vi "Actor Core.vi"(8 "error in":errorcluster, 11 "Nested in":refnum<class "ViewController.lvclass">) -> (0 "error out":errorcluster, 3 "Actor out":refnum<class "Actor.lvclass">)   [LabVIEW 2015, in "ViewController.lvlib" / "ViewController.lvclass"]
doc: "(<B>Filename</B>: Actor Framework.lvlib:Actor.lvclass:Actor Core.vi)\n\nReceives messages to the actor, reacts to them, and initiates any error handling that may shut the actor down.\n\nDescendant classes may override this VI to append parallel tasks for the actor to complete while it handles messages. Overrides use the Call Parent Method node."
uses:
  ViewController.lvclass
  <vilib>/ActorFramework/Actor/Actor.lvclass
  <vilib>/ActorFramework/Stop Msg/Stop Msg.lvclass
  Interface Messages/VI Infomation RTM Msg/VI Infomation RTM Msg.lvclass
  Interface/Interface.lvclass
  Interface Messages/VI Information Change Msg/VI Information Change Msg.lvclass
  Interface/Controls/VI Infomation.ctl
  Interface/Interface.lvlib
panel:
  in  "VI Information":T1[](array[typedef])
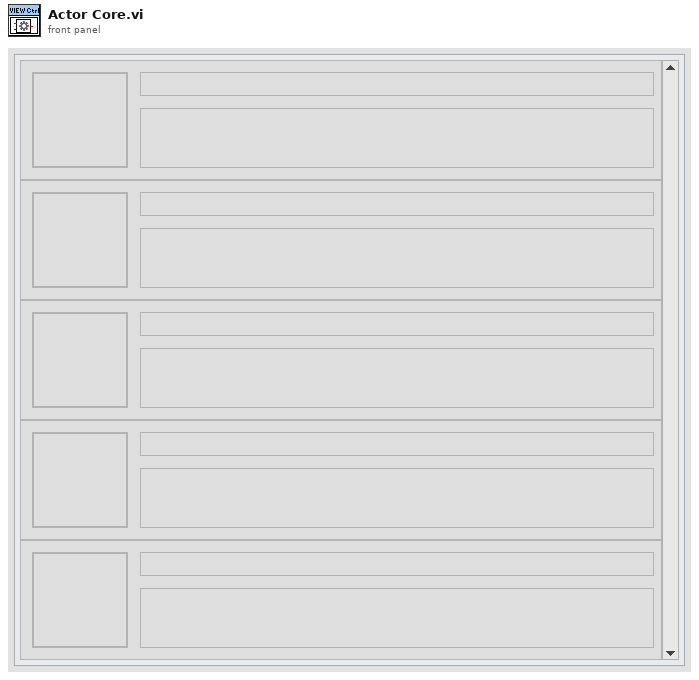
[diagram p1: front panel]
types:
  T1 = typedef "Interface.lvlib/VI Infomation.ctl" = cluster{"VI Name":string, "VI Description":string, "VI Icon":picture}
  T2 = enum8{"Enabled", "Disabled", "Disabled and Grayed Out"}
  T3 = cluster{"Stop":refnum<user-event>, "VI Infomation":refnum<user-event>}
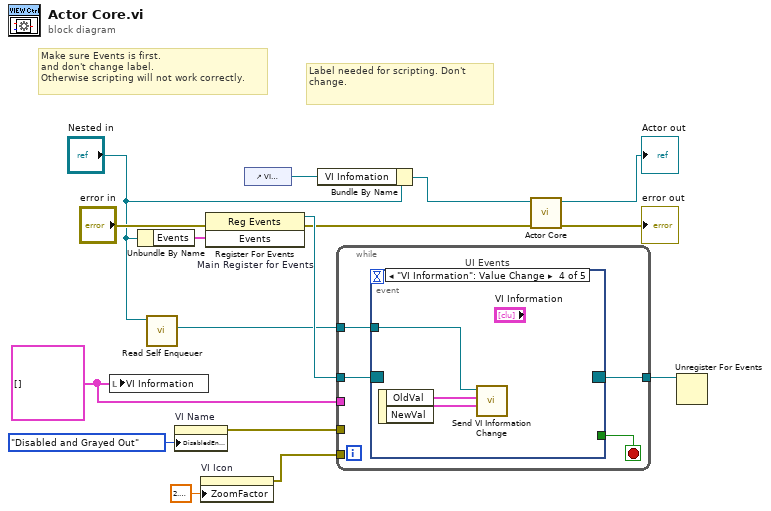
[diagram p0: block diagram]
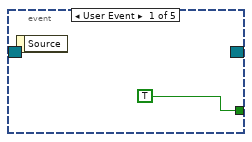
[diagram p2: hidden frame]
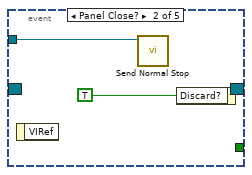
[diagram p3: hidden frame]
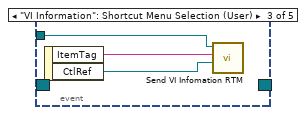
[diagram p4: hidden frame]
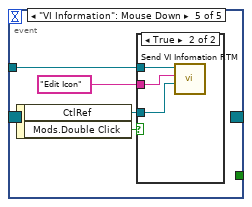
[diagram p5: hidden frame]
diagram:
  w3 = T1[] [] ("VI Information")
  # "Label needed for scripting. Don't change."
  # "Make sure Events is first.\nand don't change label.\nOtherwise scripting will not work correctly."
  n1 = local write "VI Information"(w3) -> ()
  n2 = Unbundle By Name("Nested in") -> ("Events"=w13:T3)
  n3 = call <vilib>:"Read Self Enqueuer.vi"("Actor"="Nested in") -> ("Self Enqueuer"=w11:refnum<class "Message Enqueuer.lvclass">)  [unwired: 10 in]
  n4 = property on="VI Name" class="Str"("DisabledEnum"=T2."Disabled and Grayed Out" ("Disabled")) -> (error out=w7:errorcluster)  [unwired: 2 in, 1 out]
  n5 = property on="VI Icon" class="Pict"("ZoomFactor"=sgl 2.9 ("Zoom Factor")) -> (error out=w1:errorcluster)  [unwired: 2 in, 1 out]
  n6 = register-events "Main Register for Events"(error in="error in", w13) -> (reference out=w14:refnum<event-registration>, error out=w9:errorcluster)  [unwired: 1 in]
  n7 = control-ref of="VI Information"() -> (w6:refnum<vi>)
  n8 = Bundle By Name(cluster="Nested in", "VI Infomation"=w6) -> (w4:refnum<class "ViewController.lvclass">)
  n9 = while {
    tunnel: w14 -> [w20]
    tunnel: [w18] -> w12
    tunnel: w11 -> [w17]
    tunnel: w7 -> [_]
    tunnel: w3 -> [_]
    tunnel: w1 -> [_]
    stop <- w19 stop-if-true
    n10 = event "UI Events" shown="[3] \"VI Information\": Value Change" {
      selector: w20 -> [_ _ _ _ _]
      dyn-events: [_ _ _ _ _] -> w18
      timeout: _ -> [_ _ _ _ _]
      tunnel: [TRUE _ _ _ _] -> w19
      tunnel: w17 -> [_ w22 w24 w29 w32]
      event User Event {
        n11 = event-data() -> ()  [unwired: 1 in, 1 out]
      }
      event Panel Close? {
        n12 = event-data() -> ()  [unwired: 1 in, 1 out]
        n13 = call <vilib>:"Send Normal Stop.vi"("Message Enqueuer"=w22) -> ()  [unwired: 10 in, 1 out]
        n14 = event-data("Discard?"=TRUE) -> ()  [unwired: 1 in, 1 out]
      }
      event "VI Information": Shortcut Menu Selection (User) {
        n15 = event-data() -> ("ItemTag"=w26:string, "CtlRef"=w25:refnum<vi>)  [unwired: 1 in]
        n16 = call "Send VI Infomation RTM.vi"("Ctl Refnum"=w25, "Menu Tag"=w26, "Message Enqueuer"=w24) -> ()  [unwired: 7 in, 2 out]
      }
      event "VI Information": Value Change {
        n17 = event-data() -> ("OldVal"=w28:T1[], "NewVal"=w27:T1[])  [unwired: 1 in]
        n18 = call "Send VI Information Change.vi"("New"=w27, "Old"=w28, "Message Enqueuer"=w29) -> ()  [unwired: 7 in, 2 out]
      }
      event "VI Information": Mouse Down {
        n19 = event-data() -> ("CtlRef"=w31:refnum<vi>, "Mods.Double Click"=w33:bool)  [unwired: 1 in]
        n20 = case shown="True" w33 {
          tunnel: w32 -> [_ w36]
          tunnel: w31 -> [_ w35]
          tunnel: "Edit Icon" ("Menu Tag") -> [_ w34]
          frame False {
          }
          frame True {
            n21 = call "Send VI Infomation RTM.vi"("Ctl Refnum"=w35, "Menu Tag"=w34, "Message Enqueuer"=w36) -> ()  [unwired: 7 in, 2 out]
          }
        }
      }
    }
  }
  n22 = call-parent "Actor Core.vi"("error in"=w9, "Nested in"=w4) -> ("error out"=→"error out":errorcluster, "Actor out"=→"Actor out":refnum<class "Actor.lvclass">)  [unwired: 8 in]
  n23 = Unregister For Events(event registration refnum=w12) -> ()  [unwired: 1 in, 1 out]
